vi "DELETE Handle setConfiguration.vi"(8 "error in (no error)":errorcluster, 10 "setConfiguration":variant, 11 "Inst.FP in":refnum<class "Inst.FP.lvclass">) -> (0 "error out":errorcluster, 3 "Inst.FP out":refnum<class "Inst.FP.lvclass">)   [LabVIEW 2019]
uses:
  45e4b271-6884-462c-ad3a-d505ab08eb62.vi
  Inst.FP.lvclass
  C:/Program Files (x86)/National Instruments/LabVIEW 2019/user.lib/LevyLab/Instrument Framework/Instrument Types/Cryostat/Instrument.Cryostat.lvclass
  C:/Program Files (x86)/National Instruments/LabVIEW 2019/user.lib/LevyLab/Instrument Framework/Instrument/Instrument.lvclass
  C:/Program Files (x86)/National Instruments/LabVIEW 2019/vi.lib/JKI/JKI SMO/SMO/SMO.lvclass
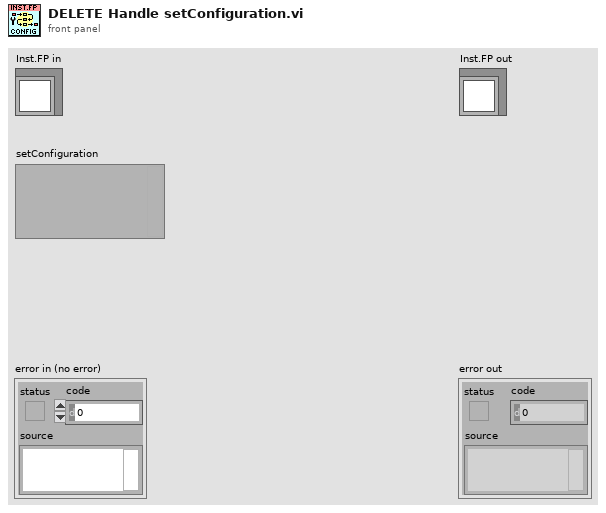
[diagram p1: front panel]
types:
  T1 = typedef "Inst.FP.lvclass/Inst.FP.Configuration--Cluster.ctl" = cluster{"FP Type":T2}
  T2 = typedef "Inst.FP.lvclass/Inst.FP.Type--Enum.ctl" = enum32{"Wet", "CF"}
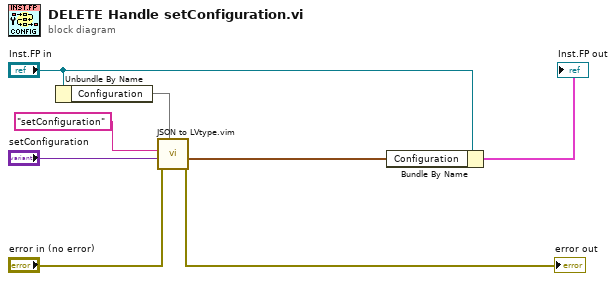
[diagram p0: block diagram]
diagram:
  n1 = Unbundle By Name("Inst.FP in") -> ("Configuration"=w7)
  n2 = call "JSON to LVtype.vim"("type"=w7, "error in (no error)"="error in (no error)", "JSON Data in"="setConfiguration", 10:"setConfiguration" ("Command")) -> ("error out"=→"error out":errorcluster, "Data out"=w1:T1)  [unwired: 6 in]
  n3 = Bundle By Name(cluster="Inst.FP in", "Configuration"=w1) -> (→"Inst.FP out":cluster{})
